vi "getArrayIndexes.vi"(11 "Array in":string[](array[string])) -> (2 "Array 2":i32[](array[numeric]), 3 "Array":i32[](array[numeric]))   [LabVIEW 2015]
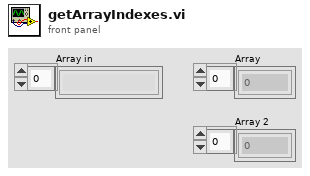
[diagram p1: front panel]
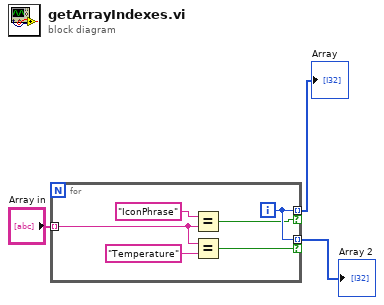
[diagram p0: block diagram]
diagram:
  n1 = for {
    tunnel: "Array in" -> [w6] mode=indexing
    tunnel: [w5] -> w1 mode=indexing if=w8
    tunnel: [w5] -> w2 mode=indexing if=w4
    i -> [w5]
    n2 = Equal?(x="IconPhrase", y=w6) -> (x = y?=w4:bool)
    n3 = Equal?(x=w6, y="Temperature") -> (x = y?=w8:bool)
  }
  "Array" <- w2
  "Array 2" <- w1
